vi "Pre Proceed Image.vi"(8 "error in (no error)":errorcluster, 11 "Display in":refnum<class "HIJ Vision Display.lvclass">) -> (0 "error out":errorcluster, 3 "Display out":refnum<class "HIJ Vision Display.lvclass">)   [LabVIEW 2014, in "HIJ Vision Display.lvlib" / "HIJ Vision Display.lvclass"]
uses:
  HIJ Vision Display.lvclass
  HIJ Vision Display.lvclass/HIJ Vision Display.ctl
  Utility/POLARIS Vision utility.lvlib
  <vilib>/vision/NI_Vision_Development_Module.lvlib
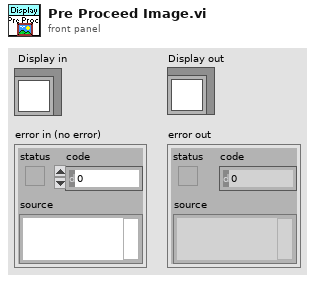
[diagram p1: front panel]
types:
  T1 = typedef "Image Type" = u32
  T2 = typedef "IMAQ Image.ctl" = refnum<image>
  T3 = typedef "ROI Descriptor" = cluster{"Global Rectangle":i32[], "Contours":cluster{"ID":enum32{"External", "Internal"}, "Type":u32, "Coordinates":i32[]}[]}
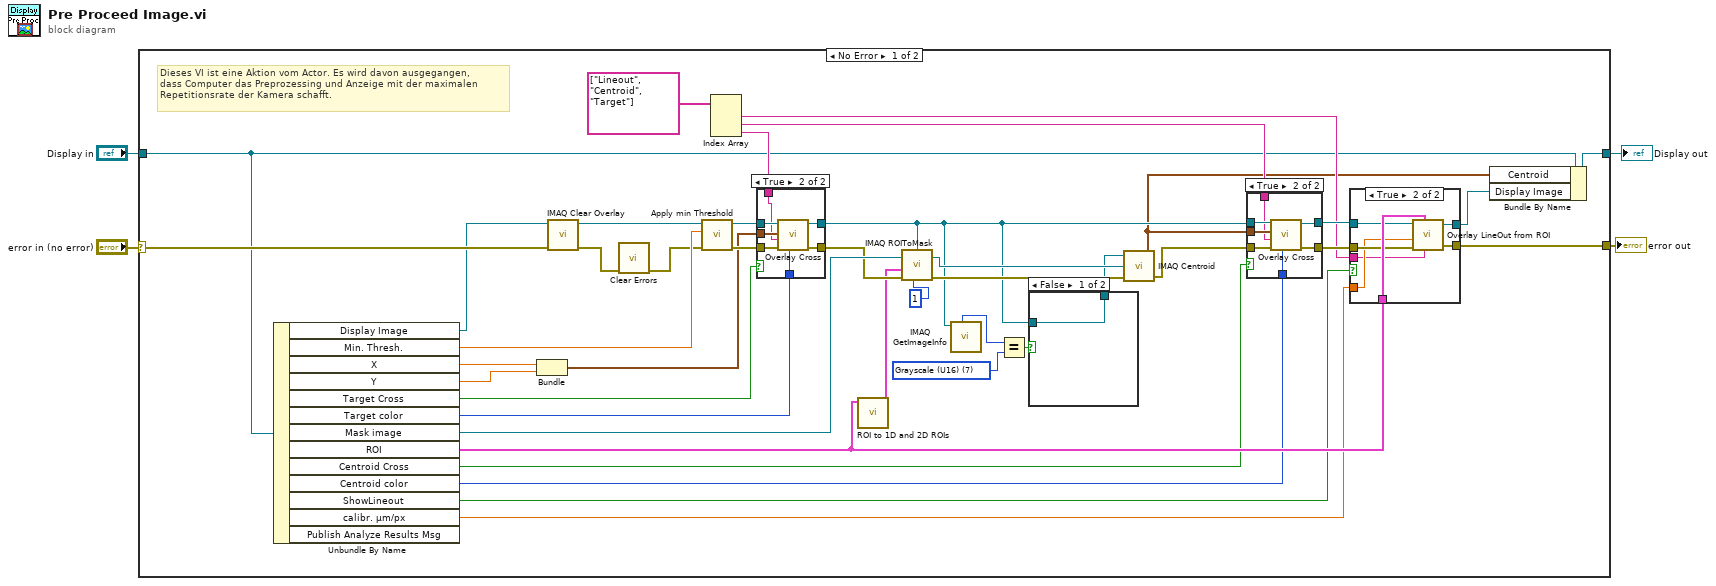
[diagram p0: block diagram]
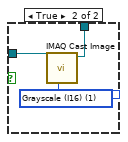
[diagram p2: hidden frame]
diagram:
  n1 = case shown="No Error" "error in (no error)" {
    selector: "error in (no error)" -> [w44 w78]
    tunnel: [w6 w78] -> w3
    tunnel: "Display in" -> [w8 w77]
    tunnel: [w7 w77] -> w1
    frame No Error {
      w19 = T1 7 items=["Grayscale (U8)", "Grayscale (I16)", "Grayscale (SGL)", "Complex (CSG)", "RGB (U32)", "HSL (U32)", "RGB (U64)", "Grayscale (U16)"] ("Image Type")
      # "Dieses VI ist eine Aktion vom Actor. Es wird davon ausgegangen,\ndass Computer das Preprozessing und Anzeige mit der maximalen\nRepetitionsrate der Kamera schafft."
      n2 = Unbundle By Name(w8) -> ("Display Image"=w11:T2, "Min. Thresh."=w24:sgl, "X"=w41:dbl, "Y"=w40:dbl, "Target Cross"=w39:bool, "Target color"=w37:u32, "Mask image"=w33:T2, "ROI"=w45:T3, "Centroid Cross"=w32:bool, "Centroid color"=w29:u32, "ShowLineout"=w26:bool, "calibr. µm/px"=w23:sgl[unit])  [unwired: 1 out]
      n3 = Bundle("X"=w41, "Y"=w40) -> (w38:cluster{"X":dbl, "Y":dbl})  [unwired: 1 in]
      n4 = call "IMAQ Clear Overlay"("error in (no error)"=w44, "Image"=w11) -> ("error out"=w10:errorcluster, "Image Out"=w25:T2)  [unwired: 8 in]
      n5 = call <vilib>:"Clear Errors.vi"("error in (no error)"=w10) -> ("error out"=w9:errorcluster)  [unwired: 5 in, 1 out]
      n6 = call "Apply min Threshold.vi"("error in"=w9, "Min. Thresh."=w24, "Image In"=w25) -> ("error out"=w42:errorcluster, "Image Out"=w43:T2)  [unwired: 7 in]
      n7 = Index Array(array=string[] ["Lineout", "Centroid", "Target"]) -> (element #1=w22:string, element #2=w21:string, element #3=w20:string)  [unwired: 3 in]
      n8 = case shown="True" w39 {
        tunnel: w43 -> [w69 w76]
        tunnel: [w69 w75] -> w13
        tunnel: w42 -> [w68 w74]
        tunnel: w38 -> [_ w73]
        tunnel: w37 -> [_ w72]
        tunnel: [w68 w71] -> w31
        tunnel: w20 -> [_ w70]
        frame False {
        }
        frame True {
          n9 = call "Overlay Cross.vi"("Color"=w72, "error in (no error)"=w74, "Overlay Group"=w70, "point"=w73, "Image In"=w76) -> ("error out"=w71:errorcluster, "Image Out"=w75:T2)  [unwired: 4 in]
        }
      }
      n10 = call "ROI to 1D and 2D ROIs.vi"("ROI Descriptor In"=w45) -> ("2D ROIs"=w15:T3)  [unwired: 9 in, 1 out]
      n11 = call "IMAQ ROIToMask"("error in (no error)"=w31, "ROI Descriptor"=w15, "Filling Value (255)"=1, "Image"=w33, "Image Model"=w13) -> ("error out"=w36:errorcluster, "Image Out"=w35:T2)  [unwired: 1 in, 1 out]
      n12 = call "IMAQ GetImageInfo"("Image"=w13) -> ("Image Type"=w18:T1)  [unwired: 3 in, 7 out]
      n13 = Equal?(x=w18, y=w19) -> (x = y?=w17:bool)
      n14 = case shown="False" w17 {
        tunnel: w13 -> [w46 w49]
        tunnel: [w46 w47] -> w16
        frame False {
        }
        frame True {
          w48 = T1 1 items=["Grayscale (U8)", "Grayscale (I16)", "Grayscale (SGL)", "Complex (CSG)", "RGB (U32)", "HSL (U32)", "RGB (U64)", "Grayscale (U16)"] ("Image Type")
          n15 = call "IMAQ Cast Image"("Image Type"=w48, "Image Src"=w49) -> ("Image Dst Out"=w47:T2)  [unwired: 8 in, 1 out]
        }
      }
      n16 = call "IMAQ Centroid"("error in (no error)"=w36, "Image Mask"=w35, "Image"=w16) -> ("error out"=w30:errorcluster, "Centroid"=w12:cluster{"X Centroid":sgl, "Y Centroid":sgl})  [unwired: 1 in]
      n17 = case shown="True" w32 {
        tunnel: w13 -> [w60 w67]
        tunnel: [w60 w66] -> w28
        tunnel: w30 -> [w59 w65]
        tunnel: w12 -> [_ w64]
        tunnel: w29 -> [_ w63]
        tunnel: [w59 w62] -> w27
        tunnel: w21 -> [_ w61]
        frame False {
        }
        frame True {
          n18 = call "Overlay Cross.vi"("Color"=w63, "error in (no error)"=w65, "Overlay Group"=w61, "point"=w64, "Image In"=w67) -> ("error out"=w62:errorcluster, "Image Out"=w66:T2)  [unwired: 4 in]
        }
      }
      n19 = case shown="True" w26 {
        tunnel: w28 -> [w51 w57]
        tunnel: w27 -> [w50 w56]
        tunnel: [w51 w55] -> w14
        tunnel: [w50 w54] -> w6
        tunnel: w23 -> [_ w53]
        tunnel: w45 -> [_ w58]
        tunnel: w22 -> [_ w52]
        frame False {
        }
        frame True {
          n20 = call "Overlay LineOut from ROI.vi"("Image In"=w57, "ROI"=w58, "Calbration"=w53, "Group"=w52, "error in"=w56) -> ("Image Out"=w55:T2, "error out"=w54:errorcluster)  [unwired: 1 in, 1 out]
        }
      }
      n21 = Bundle By Name(cluster=w8, "Centroid"=w12, "Display Image"=w14) -> (w7:refnum<class "HIJ Vision Display.lvclass">)
    }
    frame Error {
    }
  }
  "error out" <- w3
  "Display out" <- w1
